vi "Check unique part names.vi"(1 "Part IDs":string[](array[string])) -> (0 "Parts repeated":bool)   [LabVIEW 2021, in "Database Entry.lvclass"]
uses:
  Database Entry.lvclass
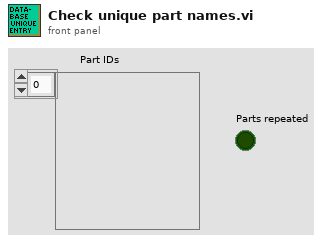
[diagram p1: front panel]
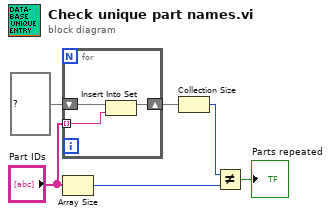
[diagram p0: block diagram]
diagram:
  n1 = for {
    tunnel: "Part IDs" -> [w8] mode=indexing
    shift-right: [w9] -> w2
    shift-left: set{string} {} ("Set") -> [w7]
    n2 = Insert Into Set(10:w8, 11:w7) -> (3:w9:set{string})  [unwired: 1 out]
  }
  n3 = Array Size(array="Part IDs") -> (size(s)=w4:i32)
  n4 = Collection Size(1:w2) -> (0:w6:i32)
  n5 = Not Equal?(x=w6, y=w4) -> (x != y?=→"Parts repeated":bool)
